vi "Move.vi"(8 "error in (no error)":errorcluster, 9 "Absolute (T)":bool=TRUE, 10 "Point":refnum<class "Point.lvclass">, 11 "Line in":refnum<class "Line.lvclass">) -> (0 "error out":errorcluster, 3 "Line out":refnum<class "Line.lvclass">)   [LabVIEW 2021, in "Picture2D.lvlib" / "Line.lvclass"]
uses:
  Line.lvclass
  Shape/Shape.lvclass
  Point/Point.lvclass
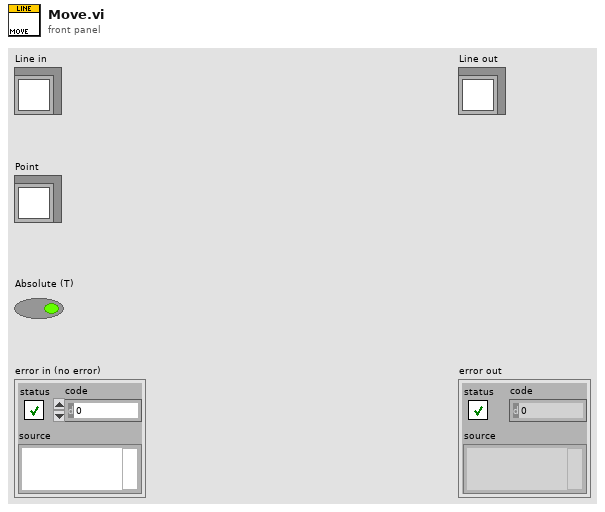
[diagram p1: front panel]
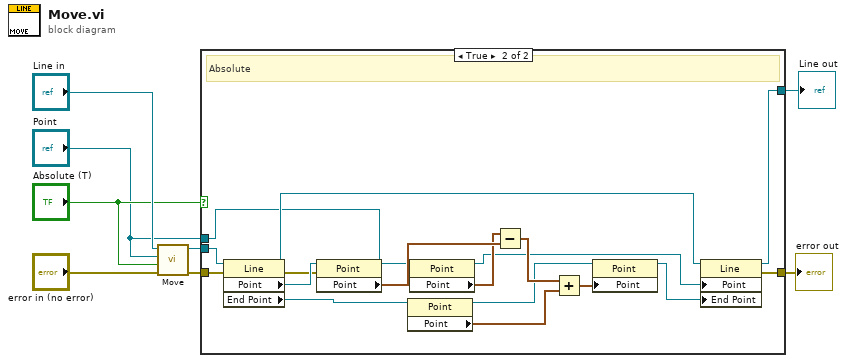
[diagram p0: block diagram]
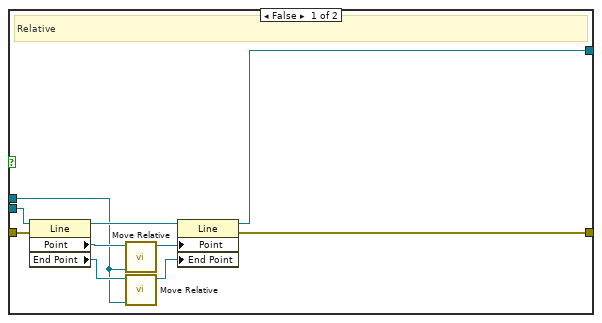
[diagram p2: hidden frame]
diagram:
  n1 = call-parent "Move.vi"("error in (no error)"="error in (no error)", "Absolute (T)"="Absolute (T)", "Point"="Point", "Shape in"="Line in") -> ("error out"=w6:errorcluster, "Shape out"=w2:refnum<class "Line.lvclass">)  [unwired: 6 in]
  n2 = case shown="True" "Absolute (T)" {
    tunnel: w6 -> [w15 w26]
    tunnel: [w14 w20] -> w5
    tunnel: "Point" -> [w10 w24]
    tunnel: w2 -> [w18 w28]
    tunnel: [w16 w29] -> w1
    frame False {
      # "Relative"
      n3 = property class="Line"(reference=w18, error in=w15) -> (reference out=w17:refnum<class "Line.lvclass">, "Point"=w13:refnum<class "Point.lvclass">, "End Point"=w11:refnum<class "Point.lvclass">)  [unwired: 1 out]
      n4 = call "Move Relative.vi"("Move"=w10, "Point"=w13) -> ("New Point"=w12:refnum<class "Point.lvclass">)  [unwired: 9 in]
      n5 = call "Move Relative.vi"("Move"=w10, "Point"=w11) -> ("New Point"=w9:refnum<class "Point.lvclass">)  [unwired: 9 in]
      n6 = property class="Line"(reference=w17, "Point"=w12, "End Point"=w9) -> (reference out=w16:refnum<class "Line.lvclass">, error out=w14:errorcluster)  [unwired: 1 in]
    }
    frame True {
      # "Absolute"
      n7 = property class="Line"(reference=w28, error in=w26) -> (reference out=w31:refnum<class "Line.lvclass">, error out=w27:errorcluster, "Point"=w35:refnum<class "Point.lvclass">, "End Point"=w22:refnum<class "Point.lvclass">)
      n8 = property class="Point"(reference=w35, error in=w27) -> ("Point"=w34:cluster{"x":i16, "y":i16})  [unwired: 2 out]
      n9 = property class="Point"(reference=w22) -> (reference out=w21:refnum<class "Point.lvclass">, "Point"=w23:cluster{"x":i16, "y":i16})  [unwired: 1 in, 1 out]
      n10 = property class="Point"(reference=w24) -> (reference out=w25:refnum<class "Point.lvclass">, "Point"=w33:cluster{"x":i16, "y":i16})  [unwired: 1 in, 1 out]
      n11 = Subtract(x=w33, y=w34) -> (x-y=w32:cluster{"x":i16, "y":i16})
      n12 = Add(x=w32, y=w23) -> (x+y=w19:cluster{"x":i16, "y":i16})
      n13 = property class="Point"(reference=w21, "Point"=w19) -> (reference out=w30:refnum<class "Point.lvclass">)  [unwired: 1 in, 1 out]
      n14 = property class="Line"(reference=w31, "Point"=w25, "End Point"=w30) -> (reference out=w29:refnum<class "Line.lvclass">, error out=w20:errorcluster)  [unwired: 1 in]
    }
  }
  "error out" <- w5
  "Line out" <- w1
